vi "20250618练习.vi"() -> ()   [LabVIEW 2024]
uses:
  <vilib>/addons/database/Auxilliary.llb/DB Tools Column Info.ctl
  <vilib>/addons/database/Auxilliary.llb/DB Tools DataTypes.ctl
  <vilib>/addons/database/Connection.llb/DB Tools Open Connec (String).vi
  <vilib>/addons/database/NI_Database_API.lvlib
  <vilib>/addons/database/Connection.llb/DB Tools Open Connec (Path).vi
panel:
  out "tables":string[](array[string])
  in  "connection information":path
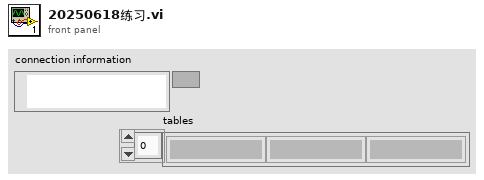
[diagram p1: front panel]
types:
  T1 = typedef "NI_Database_API.lvlib/DB Tools Column Info.ctl" = cluster{"column name":string, "data type":T2, "size":i32, "allow null?":bool}
  T2 = typedef "NI_Database_API.lvlib/DB Tools DataTypes.ctl" = enum16{"String", "Long (I32)", "Single (SGL)", "Double (DBL)", "Date/Time", "Binary"}
  T3 = typedef "NI_Database_API.lvlib/Conn ObjectReference.ctl" = refnum<k1>
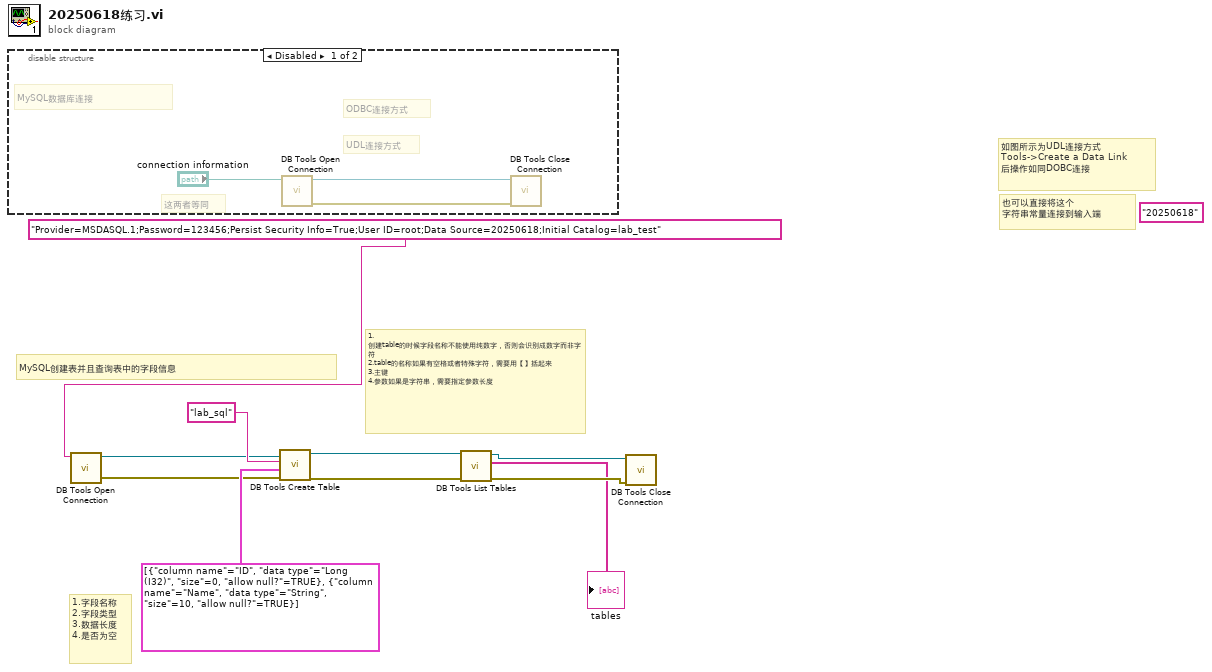
[diagram p0: block diagram]
diagram:
  (unwired) "20250618"
  # "也可以直接将这个\n字符串常量连接到输入端"
  # "如图所示为UDL连接方式\nTools->Create a Data Link\n后操作如同DOBC连接"
  # "1.创建table的时候字段名称不能使用纯数字，否则会识别成数字而非字符\n2.table的名称如果有空格或者特殊字符，需要用【】括起来\n3.主键\n4.参数如果是字符串，需要指定参数长度"
  # "1.字段名称\n2.字段类型\n3.数据长度\n4.是否为空"
  # "MySQL创建表并且查询表中的字段信息"
  n1 = disable-structure shown="Disabled" {
    frame Disabled {
      # "这两者等同"
      # "UDL连接方式"
      # "ODBC连接方式"
      # "MySQL数据库连接"
      n2 = call-poly <vilib>:"DB Tools Open Connection.vi"("connection information"="connection information") -> ("error out"=w12:errorcluster, "connection reference"=w13:T3)  [unwired: 7 in]
      n3 = call <vilib>:"DB Tools Close Connection.vi"("error in (no error)"=w12, "connection reference"=w13) -> ()  [unwired: 5 in, 1 out]
    }
    frame Enabled {
    }
  }
  n4 = call-poly <vilib>:"DB Tools Open Connection.vi"("connection information"="Provider=MSDASQL.1;Password=123456;Persist Security Info=True;User ID=root;Data Source=20250618;Initial Catalog=lab_test") -> ("error out"=w3:errorcluster, "connection reference"=w8:T3)  [unwired: 7 in]
  n5 = call <vilib>:"DB Tools Create Table.vi"("error in (no error)"=w3, "column information"=T1[] [{"column name"="ID", "data type"=enum."Long (I32)", "size"=0, "allow null?"=TRUE}, {"column name"="Name", "data type"=enum."String", "size"=10, "allow null?"=TRUE}], "table"="lab_sql", "connection reference"=w8) -> ("error out"=w4:errorcluster, "connection reference out"=w7:T3)  [unwired: 4 in]
  n6 = call <vilib>:"DB Tools List Tables.vi"("error in (no error)"=w4, "connection reference"=w7) -> ("error out"=w5:errorcluster, "tables"=→"tables":string[], "connection reference out"=w6:T3)  [unwired: 3 in]
  n7 = call <vilib>:"DB Tools Close Connection.vi"("error in (no error)"=w5, "connection reference"=w6) -> ()  [unwired: 5 in, 1 out]
